vi "wifi-receive_data.vi"(5 "error in (no error)":errorcluster, 11 "Receive bytes one time":i32, 12 "data8存盘":bool=TRUE) -> (4 "timeout?":bool, 6 "error out":errorcluster)   [LabVIEW 2023, in "wifi-interface.lvlib"]
uses:
  wifi-interface.lvlib
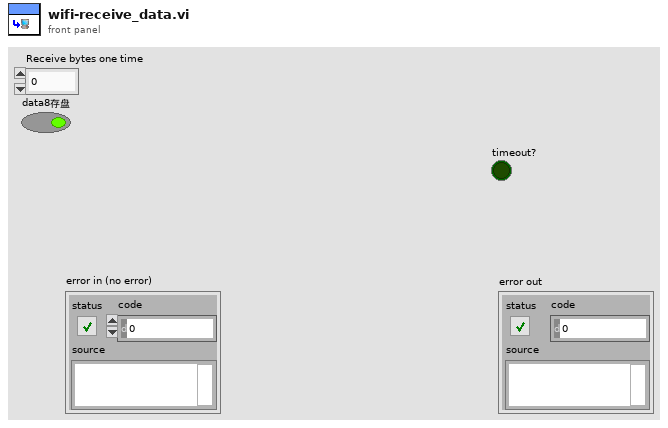
[diagram p1: front panel]
types:
  T1 = enum16{"init", "broadcast_data", "receive_data", "close", "clear_visa"}
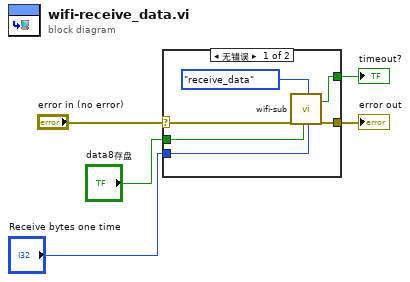
[diagram p0: block diagram]
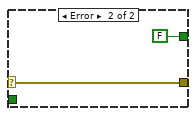
[diagram p2: hidden frame]
diagram:
  n1 = case shown="无错误" "error in (no error)" {
    selector: "error in (no error)" -> [w6 w13]
    tunnel: [w7 w13] -> w4
    tunnel: [w8 FALSE ("timeout?")] -> w3
    tunnel: "Receive bytes one time" -> [w10 _]
    tunnel: "data8存盘" -> [w9 _]
    frame No Error {
      n2 = call "wifi-sub.vi"("error in (no error)"=w6, "data存盘"=w9, "mode"=T1."receive_data", "Receive bytes one time"=w10) -> ("timeout?"=w8:bool, "error IO"=w7:errorcluster)  [unwired: 14 in]
    }
    frame Error {
    }
  }
  "error out" <- w4
  "timeout?" <- w3
